vi "Array Max & Min String Value.vi"(7 "JSON Array":refnum<class "JSON Helper.lvclass">, 11 "error in (no error)":errorcluster) -> (4 "max value":string, 6 "max index":i32, 8 "min value":string, 10 "min index":i32, 15 "error out":errorcluster)   [LabVIEW 2016]
uses:
  JSON Helper/JSON Helper.lvclass
  JSON String/Read value as String.vi
  JSON String/JSON String.lvclass
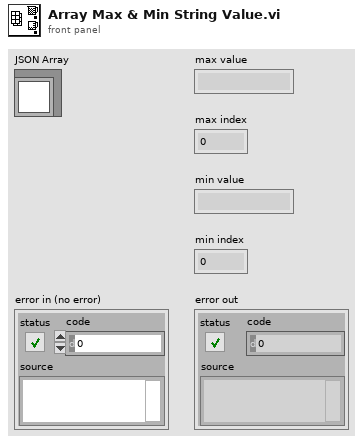
[diagram p1: front panel]
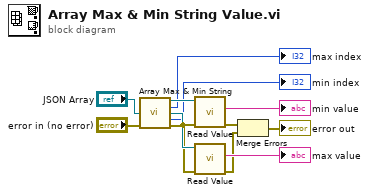
[diagram p0: block diagram]
diagram:
  n1 = call "Array Max & Min String.vi"("JSON Array"="JSON Array", "error in (no error)"="error in (no error)") -> ("max value"=w10:refnum<class "JSON String.lvclass">, "max index"=→"max index":i32, "min value"=w9:refnum<class "JSON String.lvclass">, "min index"=→"min index":i32, "error out"=w1:errorcluster)  [unwired: 9 in]
  n2 = call-poly "Read Value.vi"("error in (no error)"=w1, "JSON String in"=w10) -> ("error out"=w4:errorcluster, "value"=→"min value":string)  [unwired: 8 in]
  n3 = call-poly "Read Value.vi"("error in (no error)"=w1, "JSON String in"=w9) -> ("error out"=w3:errorcluster, "value"=→"max value":string)  [unwired: 8 in]
  n4 = Merge Errors(w4, w3) -> (→"error out":errorcluster)
